vi "Multiline_string_to_array.vi"(11 "Input string":string) -> (2 "Token positions":i32[](array[numeric]), 3 "String Array Out":string[](array[string]), 4 "LF found?":bool, 5 "Number of LF matches":i32)   [LabVIEW 2019]
uses:
  <vilib>/regexp/Match Regular Expression.xnode
panel:
  out "Str arr lengths":i32[](array[numeric])
  out "Token positions":i32[](array[numeric])
  out "String Array Out 2":string[](array[string])
  out "Substring before match array":string[](array[string])
  out "Input string length":i32
  out "offset past token":i32
  out "substring before match":string
  # "cmd.exe                    17160 Console                 0      3,196 K Running         GS66-BAMXP2\\shutters"
  # "Old programming/obsolete? (While loop at the bottom)"
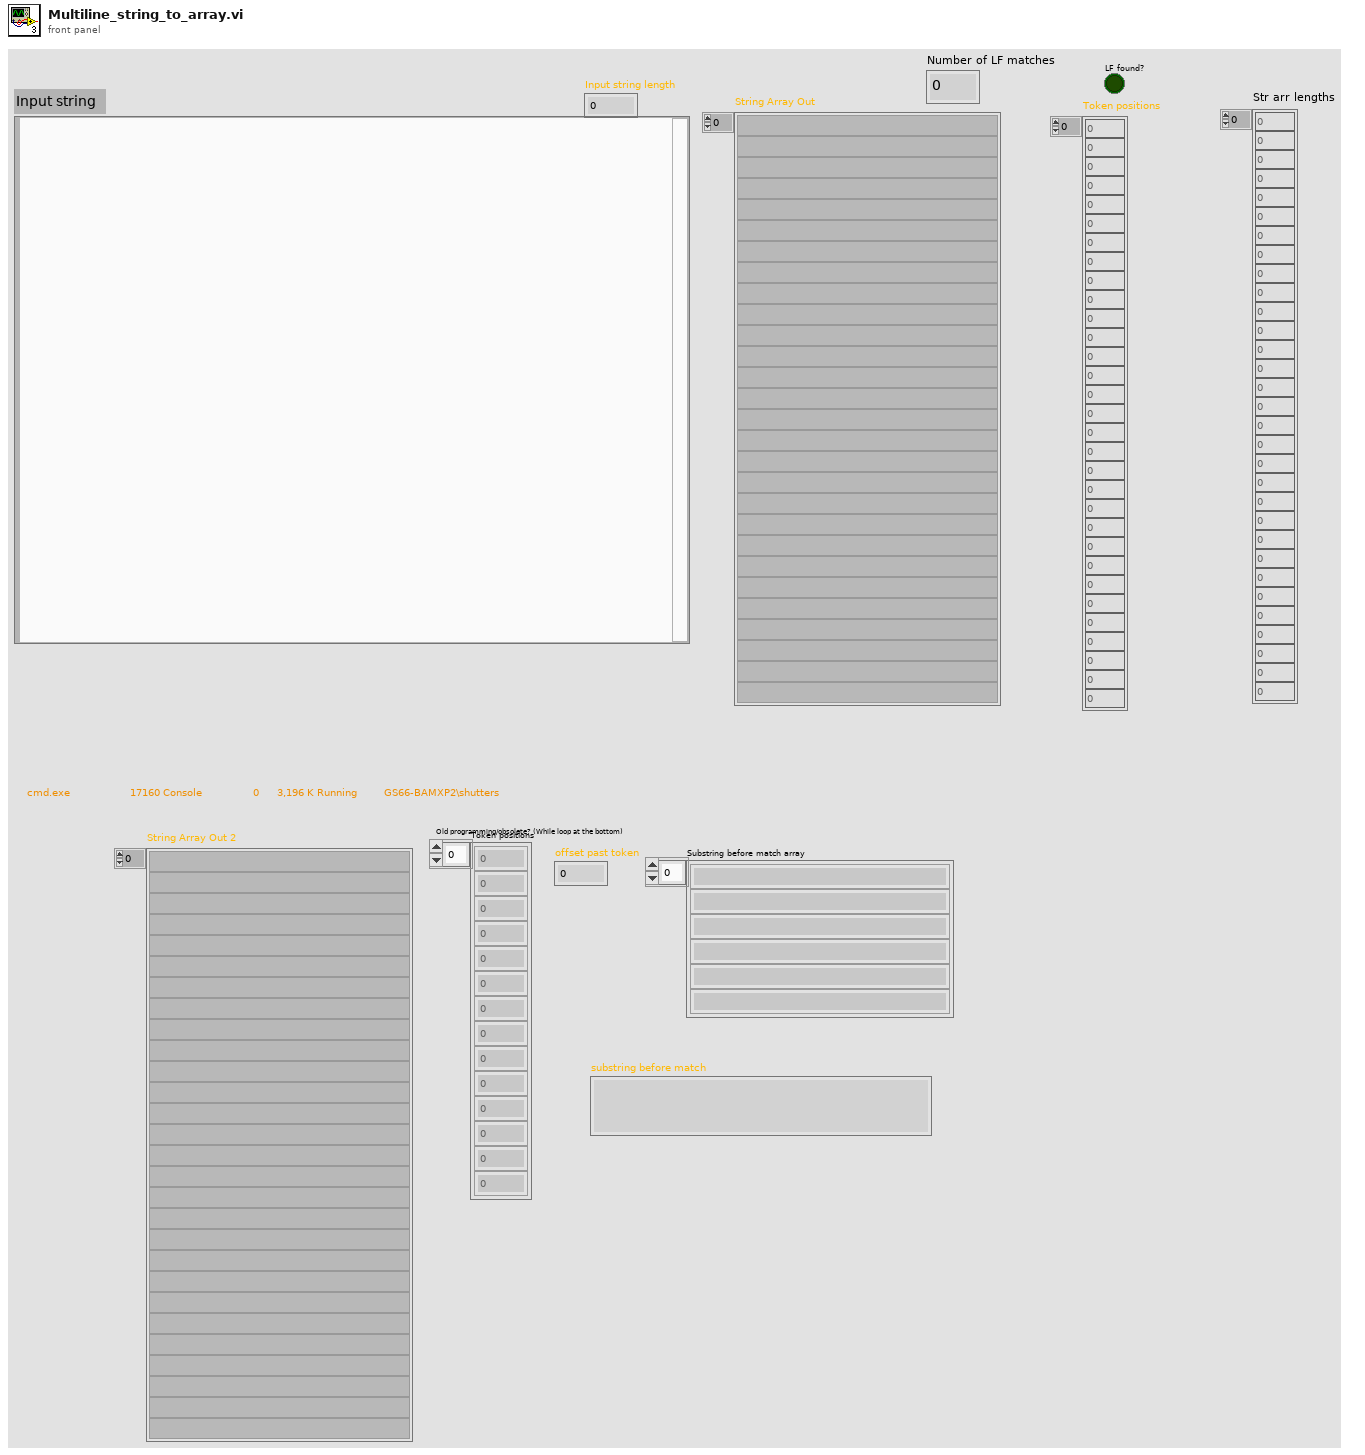
[diagram p1: front panel]
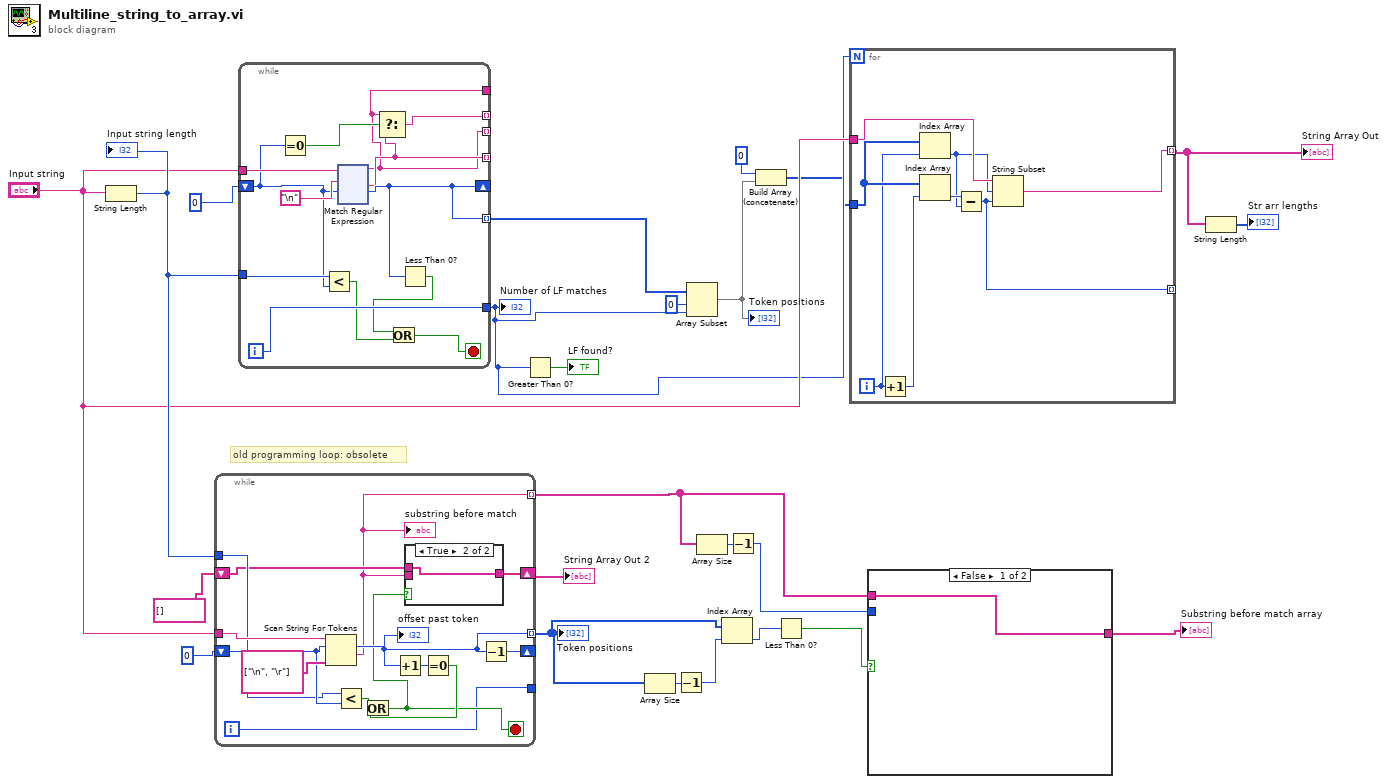
[diagram p0: block diagram]
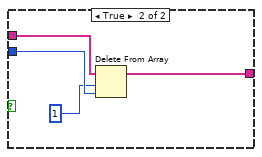
[diagram p2: hidden frame]
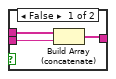
[diagram p3: hidden frame]
diagram:
  # "old programming loop: obsolete"
  n1 = String Length(string="Input string") -> (length=w21:i32)
  "Input string length" <- w21
  n2 = while {
    tunnel: w21 -> [w35]
    shift-right: [w26] -> _
    shift-left: 0 ("offset past token") -> [w36]
    tunnel: "Input string" -> [w38]
    tunnel: [w31] -> w9 mode=indexing
    shift-right: [w30] -> w20
    shift-left: string[] [] -> [w29]
    tunnel: [w27] -> w2 mode=indexing
    tunnel: [w25] -> _
    i -> [w25]
    stop <- w28 stop-if-true
    n3 = Scan String For Tokens(6:string[] ["\n", "\r"] ("delimiters (\\s,\\t,\\r,\\n)"), 8:w36, 9:w38) -> (1:w27:string, 2:w31:i32)  [unwired: 3 in, 2 out]
    "substring before match" <- w27
    "offset past token" <- w31
    n4 = Less?(x=w35, y=w36) -> (x < y?=w34:bool)
    n5 = Increment(x=w31) -> (x+1=w33:i32)
    n6 = Equal To 0?(x=w33) -> (x = 0?=w32:bool)
    n7 = Or(x=w34, y=w32) -> (x .or. y?=w28:bool)
    n8 = case shown="True" w28 {
      tunnel: w27 -> [w41 _]
      tunnel: [w40 w42] -> w30
      tunnel: w29 -> [w39 w42]
      frame False {
        n9 = Build Array (concatenate)(w39, w41) -> (w40:string[])
      }
      frame True {
      }
    }
    n10 = Decrement(x=w31) -> (x-1=w26:i32)
  }
  "String Array Out 2" <- w20
  "Token positions" <- w9
  n11 = while {
    tunnel: "Input string" -> [w55]
    shift-right: [w52] -> _
    shift-left: 0 ("offset past token") -> [w44]
    tunnel: [w51] -> _ mode=indexing
    tunnel: [w48] -> _ mode=indexing
    tunnel: [w53] -> w15
    tunnel: [w52] -> w19 mode=indexing
    tunnel: [w49] -> _ mode=indexing
    tunnel: [w48] -> _
    tunnel: w21 -> [w45]
    i -> [w53]
    stop <- w47 stop-if-true
    n12 = Equal To 0?(x=w44) -> (x = 0?=w50:bool)
    n13 = Less?(x=w45, y=w44) -> (x < y?=w43:bool)
    n14 = xnode "Match Regular Expression"("input string"=w55, "regular expression"="\n", "offset (0)"=w44) -> ("before match"=w48:string, "after match"=w51:string, "offset past match"=w52:i32)  [unwired: 3 in, 2 out]
    n15 = Select(t=w48, s=w50, f=w51) -> (s? t:f=w49:string)
    n16 = Less Than 0?(x=w52) -> (x < 0?=w46:bool)
    n17 = Or(x=w46, y=w43) -> (x .or. y?=w47:bool)
  }
  "Number of LF matches" <- w15
  n18 = Greater Than 0?(x=w15) -> (x > 0?=→"LF found?":bool)
  n19 = Array Size(array=w9) -> (size(s)=w8:i32)
  n20 = Decrement(x=w8) -> (x-1=w7:i32)
  n21 = Array Subset(array=w19, index=0, length=w15) -> (w13:i32[])
  "Token positions" <- w13
  n22 = Array Size(array=w2) -> (size(s)=w4:i32)
  n23 = Index Array(array=w9, index=w7) -> (element=w6:i32)
  n24 = Decrement(x=w4) -> (x-1=w3:i32)
  n25 = Build Array (concatenate)(0, w13) -> (w12:i32[])
  n26 = Less Than 0?(x=w6) -> (x < 0?=w5:bool)
  n27 = for {
    N: w15 -> [_]
    tunnel: "Input string" -> [w174]
    tunnel: w12 -> [w170]
    tunnel: [w172] -> w10 mode=indexing
    tunnel: [w168] -> _ mode=indexing
    i -> [w167]
    n28 = Increment(x=w167) -> (x+1=w169:i32)
    n29 = Index Array(array=w170, index=w167) -> (element=w171:i32)
    n30 = Index Array(array=w170, index=w169) -> (element=w173:i32)
    n31 = Subtract(x=w173, y=w171) -> (x-y=w168:i32)
    n32 = String Subset(string=w174, offset (0)=w171, length (rest)=w168) -> (substring=w172:string)
  }
  "String Array Out" <- w10
  n33 = case shown="False" w5 {
    tunnel: w2 -> [w175 w179]
    tunnel: w3 -> [_ w178]
    tunnel: [w175 w176] -> w1
    frame False {
    }
    frame True {
      n34 = Delete From Array(array=w179, length=1, index=w178) -> (array with subset deleted=w176:string[])  [unwired: 1 out]
    }
  }
  "Substring before match array" <- w1
  n35 = String Length(string=w10) -> (length=→"Str arr lengths":i32[])
